vi "Hanger.vi"(11 "Hanger Up":bool) -> (3 "Hanger Up":bool)   [LabVIEW 2012]
uses:
  <vilib>/Rock Robotics/WPI/Solenoid/Deprecated/WPI_SolenoidSetBool.vi
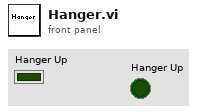
[diagram p1: front panel]
types:
  T1 = typedef "WPI_SolenoidDevRef.ctl" = cluster{"DevStatus":errorcluster, "Solenoid Module":T2, "Forward Solenoid Channel":T3, "Reverse Solenoid Channel":T3}
  T2 = typedef "FPGA_TypedefSolenoidModule.ctl" = enum16{"Solenoid Module 1", "Solenoid Module 2"}
  T3 = typedef "WPI_SolenoidChannel.ctl" = enum8{"Solenoid 1", "Solenoid 2", "Solenoid 3", "Solenoid 4", "Solenoid 5", "Solenoid 6", "Solenoid 7", "Solenoid 8", "Invalid"}
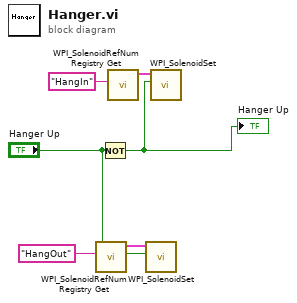
[diagram p0: block diagram]
diagram:
  n1 = call <vilib>:"WPI_SolenoidRefNum Registry Get.vi"("refnum name"="HangOut") -> ("SolenoidDevRef"=w4:T1)  [unwired: 9 in, 1 out]
  n2 = Not(x="Hanger Up") -> (.not. x?=w2:bool)
  "Hanger Up" <- w2
  n3 = call <vilib>:"WPI_SolenoidRefNum Registry Get.vi"("refnum name"="HangIn") -> ("SolenoidDevRef"=w3:T1)  [unwired: 9 in, 1 out]
  n4 = call-poly <vilib>:"WPI_SolenoidSet.vi"("Value"="Hanger Up", "SolenoidDevRef"=w4) -> ()  [unwired: 8 in, 2 out]
  n5 = call-poly <vilib>:"WPI_SolenoidSet.vi"("Value"=w2, "SolenoidDevRef"=w3) -> ()  [unwired: 8 in, 2 out]
